vi "h.ACQ.StreamFullSpectrumFromStorage.vi"(8 "error in":errorcluster, 9 "power scales and offsets":i32[][](array[numeric])=[[-60, -60, -60, -60, -60, -60, -60, -60, -60, -60, -60, -60, -60, -60, -60, -60], [1413, 1413, 1411, 1415, 1410, 1414, 1412, 1413, 1409, 1408, 1408, 1408, 1410, 1408, 1406, 1409]], 10 "Timeout":i32=10000, 11 "Connection ID In":refnum<k5>) -> (0 "error out":errorcluster, 1 "Data Available":bool, 2 "Spectral Data":T1 {"Spectrum"."Spectrum, db" format="%_8g"}, 3 "Connection ID Out":refnum<k5>)   [LabVIEW 2016, in "h.Library.lvlib"]
doc: "This VI retrieves spectral plots from a Hyperion instrument.\n\n<b>Connection ID</b> - is a network connection refnum that uniquely identifies the TCP connection\n<b>Timeout</b> - specifies the maximum amount of time, in milliseconds, for the function to complete\n<b>Channel</b> - specifies the spectrum channel number (1-16)\n<b>error in</b> - describes error conditions that occur before this node runs. This input provides standard error functionality\n<b>Connection ID out</b> - returns the same value as connection ID\n<b>Spectral Data</b> - cluster containing requested spectrum along with supporting data\n<b>error out</b> - contains error information. This output provides standard error out functionality."
uses:
  h.Library.lvlib
  CTL/h.ACQ.SpectralData.ctl
  CTL/h.ACQ.Spectrum.ctl
panel:
  # "Hyperion #StreamFullSpectrumFromStorage"
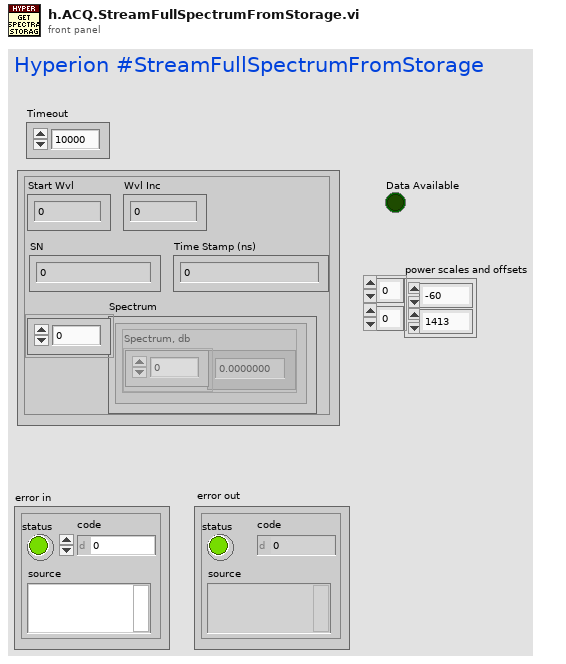
[diagram p1: front panel]
types:
  T1 = typedef "h.Library.lvlib/h.ACQ.SpectralData.ctl" = cluster{"Spectrum":T2[], "Start Wvl":dbl, "Wvl Inc":dbl, "SN":u64, "Time Stamp (ns)":u64}
  T2 = typedef "h.Library.lvlib/h.ACQ.Spectrum.ctl" = cluster{"Spectrum, db":dbl[]}
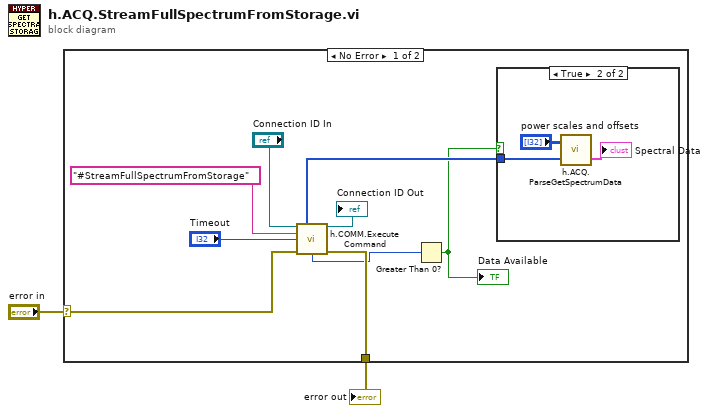
[diagram p0: block diagram]
diagram:
  n1 = case shown="No Error" "error in" {
    selector: "error in" -> [w6 w15]
    tunnel: [w5 w15] -> w1
    frame No Error {
      n2 = call "h.COMM.Execute Command.vi"("Connection ID"="Connection ID In", "Command"="#StreamFullSpectrumFromStorage", "Timeout"="Timeout", "error in"=w6) -> ("Content"=w7:u8[], "Connection ID out"=→"Connection ID Out":refnum<k5>, "Content Length"=w4:u32, "error out"=w5:errorcluster)  [unwired: 4 in, 4 out]
      n3 = Greater Than 0?(x=w4) -> (x > 0?=w3:bool)
      "Data Available" <- w3
      n4 = case shown="True" w3 {
        tunnel: w7 -> [_ w14]
        frame False {
        }
        frame True {
          n5 = call "h.ACQ.ParseGetSpectrumData.vi"("Data from #GetSpectrum"=w14, "power scales and offsets"="power scales and offsets") -> ("Spectral Data"=→"Spectral Data":T1)  [unwired: 1 in]
        }
      }
    }
    frame Error {
    }
  }
  "error out" <- w1
